vi "getSheets.vi"(8 "error in (no error)":errorcluster, 11 "MS-Excel in":refnum<class "MS-Excel.lvclass">) -> (0 "error out":errorcluster, 1 "Sheet Names":string[](array[string]), 2 "#Sheets":i32, 3 "MS-Excel out":refnum<class "MS-Excel.lvclass">)   [LabVIEW 2017, in "LabVIEW NPOI.lvlib" / "MS-Excel.lvclass"]
doc: "Protected dynamic dispatch method to get the worksheet count, in <B>#Sheet</B>, and the worksheet names list, in <B>Sheet Names</B>."
uses:
  MS-Excel.lvclass
  D:/Benjamin/Documents/Perso/Code/WC/LabVIEW_NPOI/lib/NPOI 2.1.1/NPOI.dll
  lib/NPOI 2.1.1/NPOI.dll
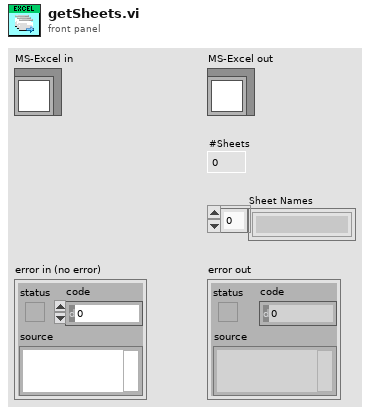
[diagram p1: front panel]
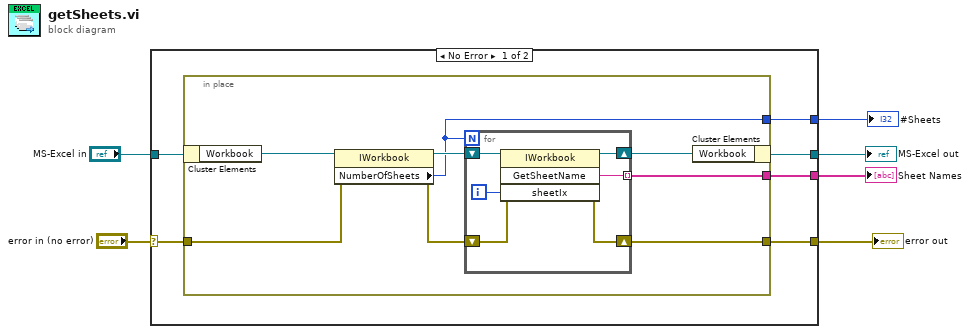
[diagram p0: block diagram]
diagram:
  n1 = case shown="No Error" "error in (no error)" {
    selector: "error in (no error)" -> [w10 w27]
    tunnel: [w9 w27] -> w6
    tunnel: [w12 w28] -> w4
    tunnel: "MS-Excel in" -> [w11 w28]
    tunnel: [w8 _] -> w2
    tunnel: [w7 _] -> w1
    frame No Error {
      n2 = in-place {
        in-place-border: w10 -> [w19]
        in-place-border: [w14] -> w9
        in-place-border: [w15] -> w8
        in-place-border: [w13] -> w7
        n3 = in-place-cluster #1(w11) -> ("Workbook"=w20:refnum<k24>)
        n4 = property class="IWorkbook"(reference=w20, error in=w19) -> (reference out=w18:refnum<k24>, error out=w17:errorcluster, "NumberOfSheets"=w15:i32)
        n5 = for {
          N: w15 -> [_]
          shift-right: [w26] -> w16
          shift-left: w18 -> [w23]
          shift-right: [w25] -> w14
          shift-left: w17 -> [w24]
          tunnel: [w21] -> w13 mode=indexing
          i -> [w22]
          n6 = invoke class="IWorkbook" method="GetSheetName"(reference=w23, error in=w24, "sheetIx"=w22) -> (reference out=w26:refnum<k24>, error out=w25:errorcluster, "GetSheetName"=w21:string)  [unwired: 1 in, 1 out]
        }
        n7 = in-place-cluster #1("Workbook"=w16) -> (w12:refnum<class "MS-Excel.lvclass">)
      }
    }
    frame Error {
    }
  }
  "error out" <- w6
  "MS-Excel out" <- w4
  "#Sheets" <- w2
  "Sheet Names" <- w1
